vi "Erase BG Color.vi"(8 "Error In":errorcluster, 11 "Table Ref In":refnum<vi>) -> (0 "Error Out":errorcluster, 3 "Table Ref Out":refnum<vi>)   [LabVIEW 2019, in "Table Tools.lvlib"]
doc: "Update Table headers."
uses:
  Table Tools.lvlib
  <vilib>/Utility/miscctls.llb/LVRowAndColumnTypeDef.ctl
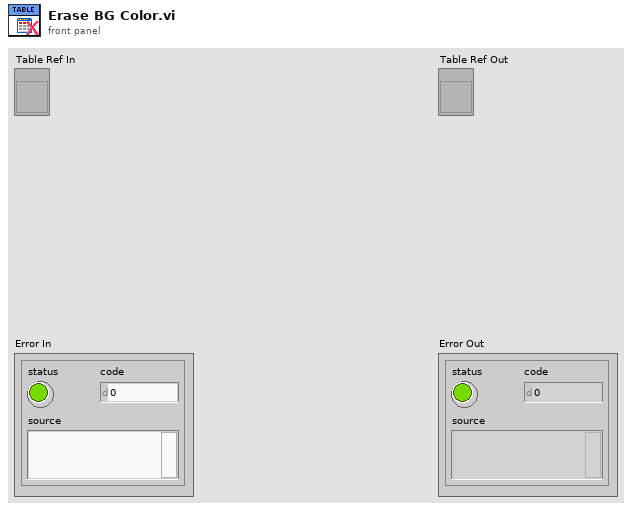
[diagram p1: front panel]
types:
  T1 = typedef "LVRowAndColumnTypeDef.ctl" = cluster{"Row":i32, "Column":i32}
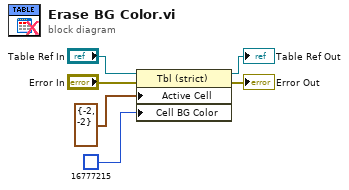
[diagram p0: block diagram]
diagram:
  n1 = property class="Tbl (strict)"(reference="Table Ref In", error in="Error In", "Active Cell"=T1 {"Row"=-2, "Column"=-2} ("Active Cell:Active Cell"), "Cell BG Color"=u32 16777215) -> (reference out=→"Table Ref Out":refnum<vi>, error out=→"Error Out":errorcluster)
